vi "test_PhotonPoseEstimator_ClosestToLastfPose.vi"(8 "error in (no error)":errorcluster) -> (0 "error out":errorcluster, 3 "Test Passed":bool)   [LabVIEW 2019]
uses:
  <vilib>/Rock Robotics/WPI/ThirdParty/JAS_Junk/TrajLib/Trajectory_Library.lvlib
  <vilib>/Rock Robotics/WPI/ThirdParty/PhotonVisionLib/PhotonVisionLib.lvlib
  <vilib>/Rock Robotics/WPI/ThirdParty/PhotonVisionLib/Enum/PhotonPoseStrategy_ENUM.ctl
  <vilib>/Rock Robotics/WPI/ThirdParty/JAS_Junk/TrajLib/TypeDef/TRANSLATION3D.ctl
  <vilib>/Rock Robotics/WPI/ThirdParty/JAS_Junk/TrajLib/TypeDef/QUATERNION.ctl
  <vilib>/Rock Robotics/WPI/ThirdParty/JAS_Junk/TrajLib/TypeDef/ROTATION3D.ctl
  <vilib>/Rock Robotics/WPI/ThirdParty/JAS_Junk/TrajLib/TypeDef/POSE3D.ctl
  <vilib>/Rock Robotics/WPI/ThirdParty/PhotonVisionLib/TypeDef/PhotonEstimatedRobotPoseType.ctl
  <vilib>/Rock Robotics/WPI/ThirdParty/PhotonVisionLib/TypeDef/TargetCornerType.ctl
  <vilib>/Rock Robotics/WPI/ThirdParty/JAS_Junk/TrajLib/TypeDef/TRANSFORM3D.ctl
  <vilib>/Rock Robotics/WPI/ThirdParty/PhotonVisionLib/TypeDef/PhotonTrackedTargetType.ctl
panel:
  out "2nd Pos Found":bool
  out "2nd Pose Est":T1={"EstimatedPose"={"Translation3d"={"X"=0.0, "Y"=0.0, "Z"=0.0}, "Rotation3d"={"Q_quaternion"={"R"=1.0, "V"=[0.0, 0.0, 0.0]}}}, "TimeStamp_Seconds"=0.0, "targetsUsed"=[], "Strategy"=enum."LOWEST_AMBIGUITY"} {"targetsUsed"."AltCameraToTarget"."TRANSLATION3D"."Z" format="%14.3f"; "targetsUsed"."AltCameraToTarget"."TRANSLATION3D"."Y" format="%14.3f"; "targetsUsed"."AltCameraToTarget"."TRANSLATION3D"."X" format="%14.3f"; "targetsUsed"."BestCameraToTarget"."TRANSLATION3D"."Z" format="%14.3f"; "targetsUsed"."BestCameraToTarget"."TRANSLATION3D"."Y" format="%14.3f"; "targetsUsed"."BestCameraToTarget"."TRANSLATION3D"."X" format="%14.3f"; "EstimatedPose"."Translation3d"."Z" format="%14.3f"; "EstimatedPose"."Translation3d"."Y" format="%14.3f"; "EstimatedPose"."Translation3d"."X" format="%14.3f"}
  out "1st Pos Found":bool
  out "1st Pose Est":T1={"EstimatedPose"={"Translation3d"={"X"=0.0, "Y"=0.0, "Z"=0.0}, "Rotation3d"={"Q_quaternion"={"R"=1.0, "V"=[0.0, 0.0, 0.0]}}}, "TimeStamp_Seconds"=0.0, "targetsUsed"=[], "Strategy"=enum."LOWEST_AMBIGUITY"} {"targetsUsed"."AltCameraToTarget"."TRANSLATION3D"."Z" format="%14.3f"; "targetsUsed"."AltCameraToTarget"."TRANSLATION3D"."Y" format="%14.3f"; "targetsUsed"."AltCameraToTarget"."TRANSLATION3D"."X" format="%14.3f"; "targetsUsed"."BestCameraToTarget"."TRANSLATION3D"."Z" format="%14.3f"; "targetsUsed"."BestCameraToTarget"."TRANSLATION3D"."Y" format="%14.3f"; "targetsUsed"."BestCameraToTarget"."TRANSLATION3D"."X" format="%14.3f"; "EstimatedPose"."Translation3d"."Z" format="%14.3f"; "EstimatedPose"."Translation3d"."Y" format="%14.3f"; "EstimatedPose"."Translation3d"."X" format="%14.3f"}
  out "Test 0 Passed":bool
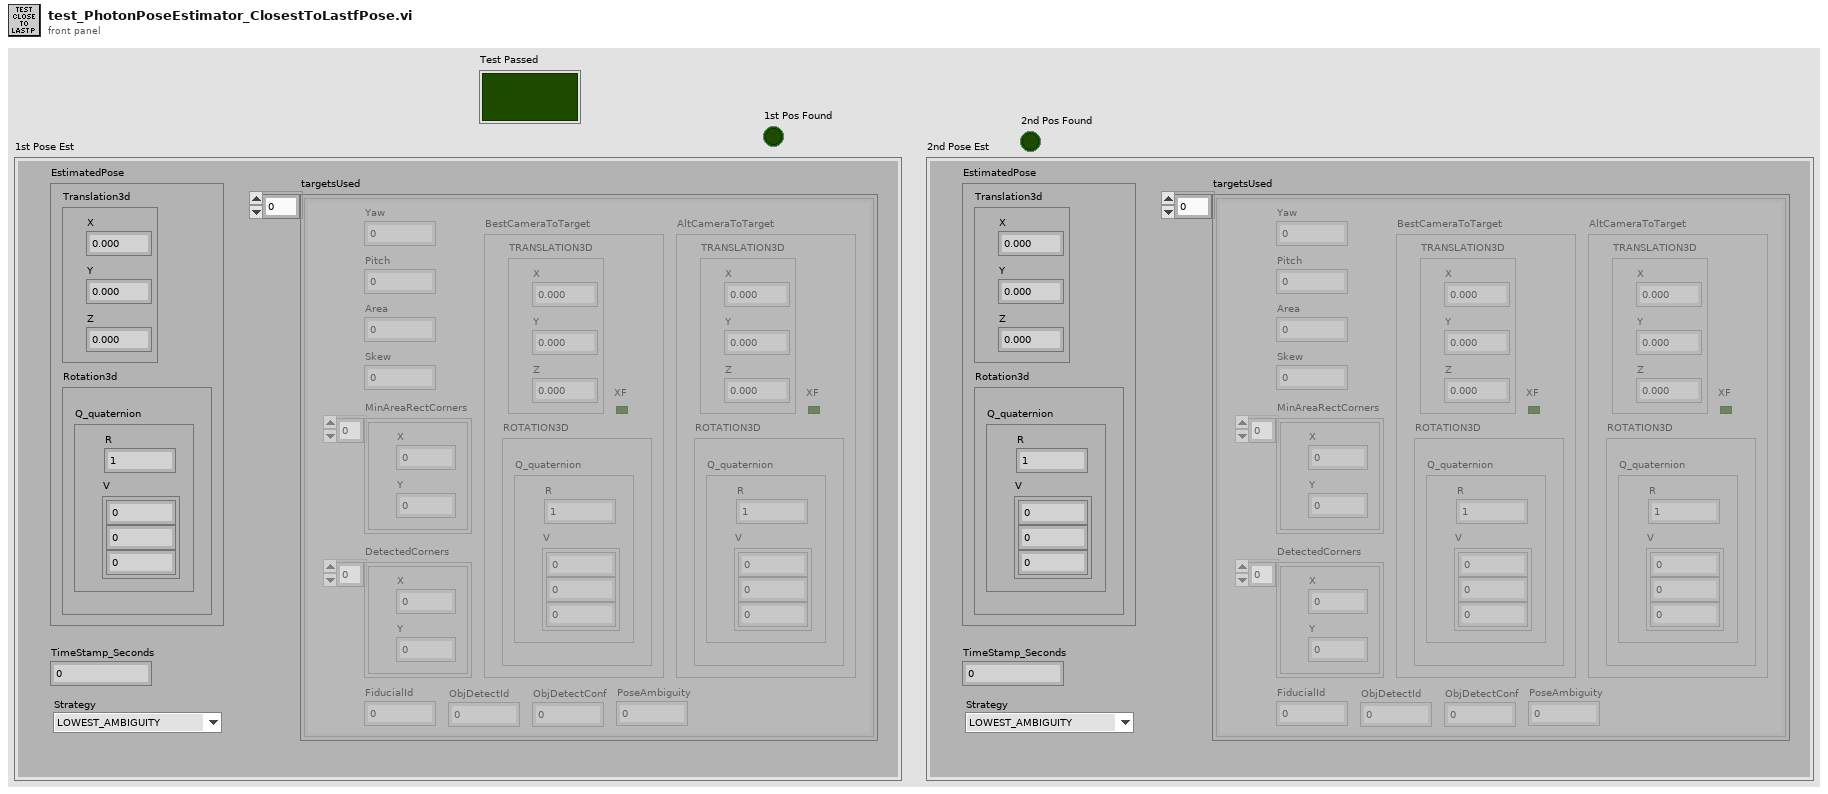
[diagram p1: front panel]
types:
  T1 = typedef "PhotonVisionLib.lvlib/PhotonEstimatedRobotPoseType.ctl" = cluster{"EstimatedPose":T2, "TimeStamp_Seconds":dbl, "targetsUsed":T6[], "Strategy":T9}
  T2 = typedef "Trajectory_Library.lvlib/POSE3D.ctl" = cluster{"Translation3d":T3, "Rotation3d":T4}
  T3 = typedef "Trajectory_Library.lvlib/TRANSLATION3D.ctl" = cluster{"X":dbl, "Y":dbl, "Z":dbl}
  T4 = typedef "Trajectory_Library.lvlib/ROTATION3D.ctl" = cluster{"Q_quaternion":T5}
  T5 = typedef "Trajectory_Library.lvlib/QUATERNION.ctl" = cluster{"R":dbl, "V":dbl[]}
  T6 = typedef "PhotonVisionLib.lvlib/PhotonTrackedTargetType.ctl" = cluster{"Yaw":dbl, "Pitch":dbl, "Area":dbl, "Skew":dbl, "MinAreaRectCorners":T7[], "BestCameraToTarget":T8, "FiducialId":i32, "AltCameraToTarget":T8, "PoseAmbiguity":dbl, "DetectedCorners":T7[], "ObjDetectId":i32, "ObjDetectConf":sgl}
  T7 = typedef "PhotonVisionLib.lvlib/TargetCornerType.ctl" = cluster{"X":dbl, "Y":dbl}
  T8 = typedef "Trajectory_Library.lvlib/TRANSFORM3D.ctl" = cluster{"TRANSLATION3D":T3, "ROTATION3D":T4, "XF":bool}
  T9 = typedef "PhotonVisionLib.lvlib/PhotonPoseStrategy_ENUM.ctl" = enum16{"LOWEST_AMBIGUITY", "CLOSEST_TO_CAMERA_HEIGHT", "CLOSEST_TO_REFERENCE_POSE", "CLOSEST_TO_LAST_POSE", "AVERAGE_BEST_TARGETS", "MULTI_TAG_PNP_ON_COPROCESSOR", "MULTI_TAG_PNP_ON_RIO"}
  T10 = typedef "Trajectory_Library.lvlib/AprilTagFieldLayout.ctl" = cluster{"AprilTagMap":map{i32, T11}, "FieldLength":dbl, "FieldWidth":dbl, "OriginPosition ":T12, "OriginPose3d":T2}
  T11 = typedef "Trajectory_Library.lvlib/AprilTag.ctl" = cluster{"ID":i32, "POSE3D":T2}
  T12 = typedef "Trajectory_Library.lvlib/AprilTagFieldLayoutOrignPosition_ENUM.ctl" = enum16{"kBlueAllianceWallRightSide,", "kRedAllianceWallRightSide,"}
  T13 = typedef "PhotonVisionLib.lvlib/PhotonPipelineMetadataType.ctl" = cluster{"CaptureTimestampMicros":i64, "PublishTimestampMicros":i64, "SequenceID":i64, "TimeSinceLastPong":i64}
  T14 = typedef "PhotonVisionLib.lvlib/PhotonPipelineResultType.ctl" = cluster{"Targets":T6[], "PhotonMultiTargetPNPResult":T15, "PhotonPipelineMetadata":T13}
  T15 = typedef "PhotonVisionLib.lvlib/PhotonMultiTargetPNPResultType.ctl" = cluster{"PhotonPNPResult":T16, "FiducialIDsUsed":i16[]}
  T16 = typedef "PhotonVisionLib.lvlib/PhotonPNPResultType.ctl" = cluster{"IsPresent":bool, "bestReprojErr":dbl, "altReprojErr":dbl, "ambiguity":dbl, "Best":T8, "Alt":T8}
  T17 = typedef "PhotonVisionLib.lvlib/PhotonPoseEstimatorType.ctl" = cluster{"LastPose":T2, "ReferencePose":T2, "FieldTags":T10, "PrimaryStratety":T9, "Camera":string, "RobotToCamera":T8, "ReportedErrors":dbl[], "HighestAmbiguity":dbl, "MultiTagFallbackStrategy":T9, "PoseCacheTimeoutSec":dbl, "PhotonTargetModel":T18, "BaseNTName":string}
  T18 = typedef "PhotonVisionLib.lvlib/PhotonTargetModel.ctl" = cluster{"Vertices":T3[], "IsPlaner":bool, "IsSpherical":bool}
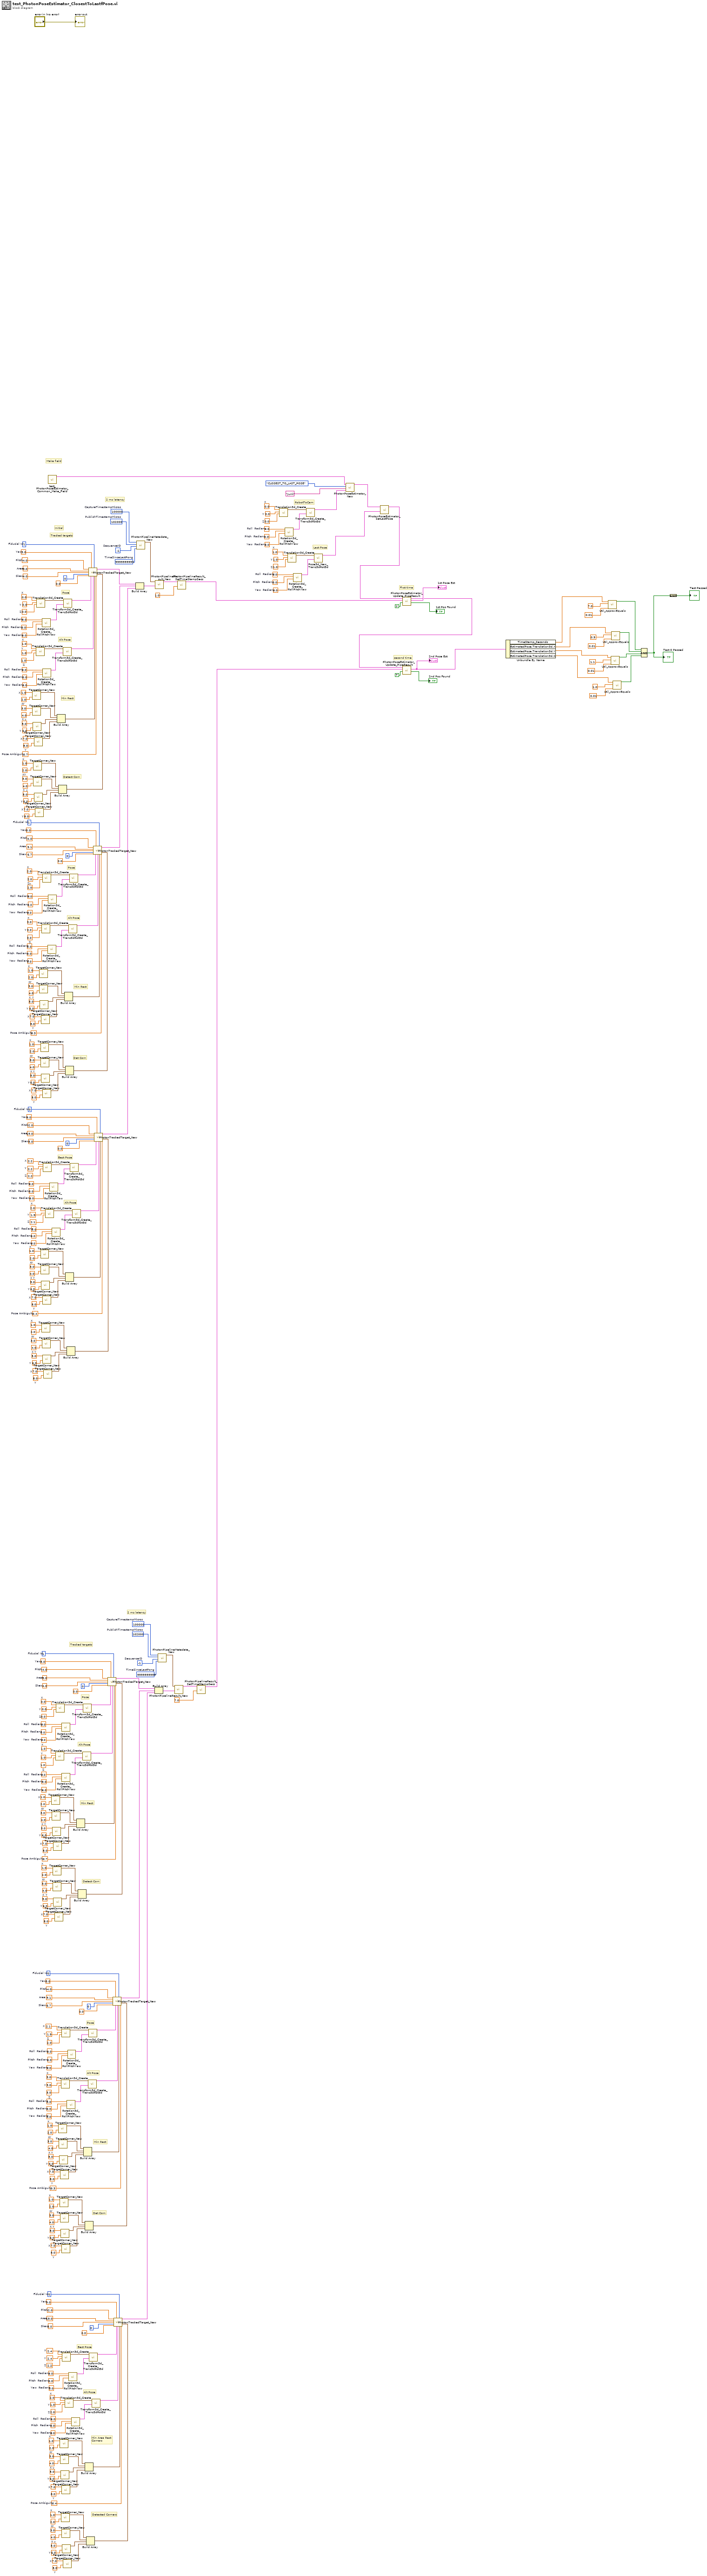
[diagram p0: block diagram]
diagram:
  w15 = i64 100000  # CaptureTimestampMicros
  w16 = i64 102000  # PublishTimestampMicros
  w17 = i64 -1  # SequenceID
  w18 = i64 9999999999  # TimeSinceLastPong
  w20 = i64 100000  # CaptureTimestampMicros
  w21 = i64 102000  # PublishTimestampMicros
  w22 = i64 -1  # SequenceID
  w23 = i64 9999999999  # TimeSinceLastPong
  w46 = 0.0  # Roll  Radians
  w45 = 0.0  # Pitch  Radians
  w44 = 0.0  # Yaw  Radians
  w49 = 2.2  # Z
  w48 = 2.4  # X
  w47 = 2.4  # Y
  w54 = 0.0  # Roll  Radians
  w53 = 0.0  # Pitch  Radians
  w52 = 0.0  # Yaw  Radians
  w57 = 2.0  # Z
  w56 = 2.0  # X
  w55 = 1.0  # Y
  w64 = 7.0  # X
  w65 = 8.0  # Y
  w66 = 5.0  # X
  w67 = 6.0  # Y
  w68 = 3.0  # X
  w69 = 4.0  # Y
  w70 = 1.0  # X
  w71 = 2.0  # Y
  w76 = 7.0  # X
  w77 = 8.0  # Y
  w78 = 5.0  # X
  w79 = 6.0  # Y
  w80 = 3.0  # X
  w81 = 4.0  # Y
  w82 = 1.0  # X
  w83 = 2.0  # Y
  w84 = -2.0  # Pitch
  w85 = 19.0  # Area
  w86 = 3.0  # Skew
  w87 = 0  # Fiducial Id
  w88 = 0.4  # Pose Ambiguity
  w89 = 9.0  # Yaw
  w96 = 0.0  # Roll  Radians
  w95 = 0.0  # Pitch  Radians
  w94 = 0.0  # Yaw  Radians
  w99 = 2.0  # Z
  w98 = 2.1  # X
  w97 = 1.9  # Y
  w104 = 0.0  # Roll  Radians
  w103 = 0.0  # Pitch  Radians
  w102 = 0.0  # Yaw  Radians
  w107 = 3.0  # Z
  w106 = 3.0  # X
  w105 = 3.0  # Y
  w114 = 7.0  # X
  w115 = 8.0  # Y
  w116 = 5.0  # X
  w117 = 6.0  # Y
  w118 = 3.0  # X
  w119 = 4.0  # Y
  w120 = 1.0  # X
  w121 = 2.0  # Y
  w126 = 7.0  # X
  w127 = 8.0  # Y
  w128 = 5.0  # X
  w129 = 6.0  # Y
  w130 = 3.0  # X
  w131 = 4.0  # Y
  w132 = 1.0  # X
  w133 = 2.0  # Y
  w134 = -4.0  # Pitch
  w135 = 9.1  # Area
  w136 = 6.7  # Skew
  w137 = 0  # Fiducial Id
  w138 = 0.3  # Pose Ambiguity
  w139 = 3.0  # Yaw
  w145 = 0.0  # Roll  Radians
  w144 = 0.0  # Pitch  Radians
  w143 = 0.0  # Yaw  Radians
  w148 = 0.0  # Z
  w147 = 0.0  # X
  w146 = 0.0  # Y
  w153 = 0.0  # Roll  Radians
  w152 = 0.0  # Pitch  Radians
  w151 = 0.0  # Yaw  Radians
  w156 = 1.0  # Z
  w155 = 1.0  # X
  w154 = 1.0  # Y
  w163 = 7.0  # X
  w164 = 8.0  # Y
  w165 = 5.0  # X
  w166 = 6.0  # Y
  w167 = 3.0  # X
  w168 = 4.0  # Y
  w169 = 1.0  # X
  w170 = 2.0  # Y
  w175 = 7.0  # X
  w176 = 8.0  # Y
  w177 = 5.0  # X
  w178 = 6.0  # Y
  w179 = 3.0  # X
  w180 = 4.0  # Y
  w181 = 1.0  # X
  w182 = 2.0  # Y
  w183 = -4.0  # Pitch
  w184 = 9.0  # Area
  w185 = 4.0  # Skew
  w186 = 1  # Fiducial Id
  w187 = 0.7  # Pose Ambiguity
  w188 = 3.0  # Yaw
  w194 = 0.0  # Roll  Radians
  w193 = 0.0  # Pitch  Radians
  w192 = 0.0  # Yaw  Radians
  w197 = 1.0  # Z
  w196 = 1.0  # X
  w195 = 1.0  # Y
  w208 = 0.0  # Roll  Radians
  w207 = 0.0  # Pitch  Radians
  w206 = 0.0  # Yaw  Radians
  w211 = 0.0  # Z
  w210 = 0.0  # X
  w209 = 0.0  # Y
  w236 = 0.0  # Roll  Radians
  w235 = 0.0  # Pitch  Radians
  w234 = 0.0  # Yaw  Radians
  w239 = 2.2  # Z
  w238 = 2.2  # X
  w237 = 2.2  # Y
  w244 = 0.0  # Roll  Radians
  w243 = 0.0  # Pitch  Radians
  w242 = 0.0  # Yaw  Radians
  w247 = 2.1  # Z
  w246 = 2.0  # X
  w245 = 1.9  # Y
  w254 = 7.0  # X
  w255 = 8.0  # Y
  w256 = 5.0  # X
  w257 = 6.0  # Y
  w258 = 3.0  # X
  w259 = 4.0  # Y
  w260 = 1.0  # X
  w261 = 2.0  # Y
  w266 = 7.0  # X
  w267 = 8.0  # Y
  w268 = 5.0  # X
  w269 = 6.0  # Y
  w270 = 3.0  # X
  w271 = 4.0  # Y
  w272 = 1.0  # X
  w273 = 2.0  # Y
  w274 = -2.0  # Pitch
  w275 = 19.0  # Area
  w276 = 3.0  # Skew
  w277 = 0  # Fiducial Id
  w278 = 0.4  # Pose Ambiguity
  w279 = 9.0  # Yaw
  w286 = 0.0  # Roll  Radians
  w285 = 0.0  # Pitch  Radians
  w284 = 0.0  # Yaw  Radians
  w289 = 2.0  # Z
  w288 = 2.0  # X
  w287 = 2.0  # Y
  w294 = 0.0  # Roll  Radians
  w293 = 0.0  # Pitch  Radians
  w292 = 0.0  # Yaw  Radians
  w297 = 3.0  # Z
  w296 = 3.0  # X
  w295 = 3.0  # Y
  w304 = 7.0  # X
  w305 = 8.0  # Y
  w306 = 5.0  # X
  w307 = 6.0  # Y
  w308 = 3.0  # X
  w309 = 4.0  # Y
  w310 = 1.0  # X
  w311 = 2.0  # Y
  w316 = 7.0  # X
  w317 = 8.0  # Y
  w318 = 5.0  # X
  w319 = 6.0  # Y
  w320 = 3.0  # X
  w321 = 4.0  # Y
  w322 = 1.0  # X
  w323 = 2.0  # Y
  w324 = -4.0  # Pitch
  w325 = 9.1  # Area
  w326 = 6.7  # Skew
  w327 = 1  # Fiducial Id
  w328 = 0.3  # Pose Ambiguity
  w329 = 3.0  # Yaw
  w336 = 0.0  # Roll  Radians
  w335 = 0.0  # Pitch  Radians
  w334 = 0.0  # Yaw  Radians
  w339 = 0.0  # Z
  w338 = 0.0  # X
  w337 = 0.0  # Y
  w344 = 0.0  # Roll  Radians
  w343 = 0.0  # Pitch  Radians
  w342 = 0.0  # Yaw  Radians
  w347 = 1.0  # Z
  w346 = 1.0  # X
  w345 = 1.0  # Y
  w354 = 7.0  # X
  w355 = 8.0  # Y
  w356 = 5.0  # X
  w357 = 6.0  # Y
  w358 = 3.0  # X
  w359 = 4.0  # Y
  w360 = 1.0  # X
  w361 = 2.0  # Y
  w366 = 7.0  # X
  w367 = 8.0  # Y
  w368 = 5.0  # X
  w369 = 6.0  # Y
  w370 = 3.0  # X
  w371 = 4.0  # Y
  w372 = 1.0  # X
  w373 = 2.0  # Y
  w374 = -4.0  # Pitch
  w375 = 9.0  # Area
  w376 = 4.0  # Skew
  w377 = 1  # Fiducial Id
  w378 = 0.7  # Pose Ambiguity
  w379 = 3.0  # Yaw
  # "2 ms latency"
  # "2 ms latency"
  # "Min Area Rect\nCorners"
  # "Detected Corners"
  # "second time"
  # "First time"
  # "Initial"
  # "Det Corn"
  # "Min Rect"
  # "Pose"
  # "Detect Corn"
  # "Min Rect"
  # "Tracked targets"
  # "Best Pose"
  # "Alt Pose"
  # "Alt Pose"
  # "Pose"
  # "Alt Pose"
  # "Last Pose"
  # "RobotToCam"
  # "Det Corn"
  # "Min Rect"
  # "Pose"
  # "Detect Corn"
  # "Min Rect"
  # "Tracked targets"
  # "Make field"
  # "Best Pose"
  # "Alt Pose"
  # "Alt Pose"
  # "Pose"
  # "Alt Pose"
  n1 = call <vilib>:"TargetCorner_New.vi"("Y"=w373, "X"=w372) -> ("TargetCorner"=w365:T7)  [unwired: 9 in]
  n2 = call <vilib>:"TargetCorner_New.vi"("Y"=w371, "X"=w370) -> ("TargetCorner"=w364:T7)  [unwired: 9 in]
  n3 = call <vilib>:"TargetCorner_New.vi"("Y"=w369, "X"=w368) -> ("TargetCorner"=w363:T7)  [unwired: 9 in]
  n4 = call <vilib>:"TargetCorner_New.vi"("Y"=w361, "X"=w360) -> ("TargetCorner"=w353:T7)  [unwired: 9 in]
  n5 = call <vilib>:"TargetCorner_New.vi"("Y"=w359, "X"=w358) -> ("TargetCorner"=w352:T7)  [unwired: 9 in]
  n6 = call <vilib>:"TargetCorner_New.vi"("Y"=w367, "X"=w366) -> ("TargetCorner"=w362:T7)  [unwired: 9 in]
  n7 = call <vilib>:"TargetCorner_New.vi"("Y"=w357, "X"=w356) -> ("TargetCorner"=w351:T7)  [unwired: 9 in]
  n8 = call <vilib>:"TargetCorner_New.vi"("Y"=w355, "X"=w354) -> ("TargetCorner"=w350:T7)  [unwired: 9 in]
  n9 = call <vilib>:"Translation3d_Create.vi"("Z"=w347, "Y"=w345, "X"=w346) -> ("TRANSLATION3D"=w341:T3)  [unwired: 8 in]
  n10 = call <vilib>:"Translation3d_Create.vi"("Z"=w339, "Y"=w337, "X"=w338) -> ("TRANSLATION3D"=w333:T3)  [unwired: 8 in]
  n11 = call <vilib>:"TargetCorner_New.vi"("Y"=w323, "X"=w322) -> ("TargetCorner"=w315:T7)  [unwired: 9 in]
  n12 = call <vilib>:"TargetCorner_New.vi"("Y"=w321, "X"=w320) -> ("TargetCorner"=w314:T7)  [unwired: 9 in]
  n13 = call <vilib>:"TargetCorner_New.vi"("Y"=w319, "X"=w318) -> ("TargetCorner"=w313:T7)  [unwired: 9 in]
  n14 = call <vilib>:"TargetCorner_New.vi"("Y"=w311, "X"=w310) -> ("TargetCorner"=w303:T7)  [unwired: 9 in]
  n15 = call <vilib>:"TargetCorner_New.vi"("Y"=w273, "X"=w272) -> ("TargetCorner"=w265:T7)  [unwired: 9 in]
  n16 = call <vilib>:"TargetCorner_New.vi"("Y"=w309, "X"=w308) -> ("TargetCorner"=w302:T7)  [unwired: 9 in]
  n17 = call <vilib>:"TargetCorner_New.vi"("Y"=w271, "X"=w270) -> ("TargetCorner"=w264:T7)  [unwired: 9 in]
  n18 = call <vilib>:"TargetCorner_New.vi"("Y"=w317, "X"=w316) -> ("TargetCorner"=w312:T7)  [unwired: 9 in]
  n19 = call <vilib>:"TargetCorner_New.vi"("Y"=w307, "X"=w306) -> ("TargetCorner"=w301:T7)  [unwired: 9 in]
  n20 = call <vilib>:"TargetCorner_New.vi"("Y"=w269, "X"=w268) -> ("TargetCorner"=w263:T7)  [unwired: 9 in]
  n21 = call <vilib>:"Translation3d_Create.vi"("Z"=w297, "Y"=w295, "X"=w296) -> ("TRANSLATION3D"=w291:T3)  [unwired: 8 in]
  n22 = call <vilib>:"TargetCorner_New.vi"("Y"=w261, "X"=w260) -> ("TargetCorner"=w253:T7)  [unwired: 9 in]
  n23 = call <vilib>:"Rotation3d_Create_RollPitchYaw.vi"("Yaw"=w334, "Pitch"=w335, "Roll"=w336) -> ("Rotation3d"=w332:T4)  [unwired: 8 in]
  n24 = call <vilib>:"TargetCorner_New.vi"("Y"=w259, "X"=w258) -> ("TargetCorner"=w252:T7)  [unwired: 9 in]
  n25 = call <vilib>:"Rotation3d_Create_RollPitchYaw.vi"("Yaw"=w342, "Pitch"=w343, "Roll"=w344) -> ("Rotation3d"=w340:T4)  [unwired: 8 in]
  n26 = call <vilib>:"Translation3d_Create.vi"("Z"=w289, "Y"=w287, "X"=w288) -> ("TRANSLATION3D"=w283:T3)  [unwired: 8 in]
  n27 = call <vilib>:"TargetCorner_New.vi"("Y"=w305, "X"=w304) -> ("TargetCorner"=w300:T7)  [unwired: 9 in]
  n28 = call <vilib>:"TargetCorner_New.vi"("Y"=w267, "X"=w266) -> ("TargetCorner"=w262:T7)  [unwired: 9 in]
  n29 = call <vilib>:"TargetCorner_New.vi"("Y"=w257, "X"=w256) -> ("TargetCorner"=w251:T7)  [unwired: 9 in]
  n30 = call <vilib>:"Translation3d_Create.vi"("Z"=w239, "Y"=w237, "X"=w238) -> ("TRANSLATION3D"=w233:T3)  [unwired: 8 in]
  n31 = call <vilib>:"TargetCorner_New.vi"("Y"=w255, "X"=w254) -> ("TargetCorner"=w250:T7)  [unwired: 9 in]
  n32 = call <vilib>:"Translation3d_Create.vi"("Z"=w247, "Y"=w245, "X"=w246) -> ("TRANSLATION3D"=w241:T3)  [unwired: 8 in]
  n33 = call <vilib>:"Rotation3d_Create_RollPitchYaw.vi"("Yaw"=w292, "Pitch"=w293, "Roll"=w294) -> ("Rotation3d"=w290:T4)  [unwired: 8 in]
  n34 = call <vilib>:"Rotation3d_Create_RollPitchYaw.vi"("Yaw"=w284, "Pitch"=w285, "Roll"=w286) -> ("Rotation3d"=w282:T4)  [unwired: 8 in]
  n35 = call "test_PhotonPoseEstimator_Common_Make_Field.vi"() -> ("AprilTagFieldLayout"=w223:T10)  [unwired: 11 in]
  n36 = call <vilib>:"Rotation3d_Create_RollPitchYaw.vi"("Yaw"=w234, "Pitch"=w235, "Roll"=w236) -> ("Rotation3d"=w232:T4)  [unwired: 8 in]
  n37 = call <vilib>:"TargetCorner_New.vi"("Y"=w182, "X"=w181) -> ("TargetCorner"=w174:T7)  [unwired: 9 in]
  n38 = call <vilib>:"Rotation3d_Create_RollPitchYaw.vi"("Yaw"=w242, "Pitch"=w243, "Roll"=w244) -> ("Rotation3d"=w240:T4)  [unwired: 8 in]
  n39 = call <vilib>:"TargetCorner_New.vi"("Y"=w180, "X"=w179) -> ("TargetCorner"=w173:T7)  [unwired: 9 in]
  n40 = call <vilib>:"TargetCorner_New.vi"("Y"=w178, "X"=w177) -> ("TargetCorner"=w172:T7)  [unwired: 9 in]
  n41 = call <vilib>:"TargetCorner_New.vi"("Y"=w170, "X"=w169) -> ("TargetCorner"=w162:T7)  [unwired: 9 in]
  n42 = call <vilib>:"TargetCorner_New.vi"("Y"=w168, "X"=w167) -> ("TargetCorner"=w161:T7)  [unwired: 9 in]
  n43 = call <vilib>:"TargetCorner_New.vi"("Y"=w176, "X"=w175) -> ("TargetCorner"=w171:T7)  [unwired: 9 in]
  n44 = call <vilib>:"TargetCorner_New.vi"("Y"=w166, "X"=w165) -> ("TargetCorner"=w160:T7)  [unwired: 9 in]
  n45 = call <vilib>:"TargetCorner_New.vi"("Y"=w164, "X"=w163) -> ("TargetCorner"=w159:T7)  [unwired: 9 in]
  n46 = call <vilib>:"Translation3d_Create.vi"("Z"=w156, "Y"=w154, "X"=w155) -> ("TRANSLATION3D"=w150:T3)  [unwired: 8 in]
  n47 = call <vilib>:"Translation3d_Create.vi"("Z"=w148, "Y"=w146, "X"=w147) -> ("TRANSLATION3D"=w142:T3)  [unwired: 8 in]
  n48 = Build Array(w365, w364, w363, w362) -> (w349:T7[])
  n49 = Build Array(w353, w352, w351, w350) -> (w348:T7[])
  n50 = call <vilib>:"TargetCorner_New.vi"("Y"=w133, "X"=w132) -> ("TargetCorner"=w125:T7)  [unwired: 9 in]
  n51 = call <vilib>:"TargetCorner_New.vi"("Y"=w131, "X"=w130) -> ("TargetCorner"=w124:T7)  [unwired: 9 in]
  n52 = call <vilib>:"TargetCorner_New.vi"("Y"=w129, "X"=w128) -> ("TargetCorner"=w123:T7)  [unwired: 9 in]
  n53 = call <vilib>:"TargetCorner_New.vi"("Y"=w121, "X"=w120) -> ("TargetCorner"=w113:T7)  [unwired: 9 in]
  n54 = call <vilib>:"TargetCorner_New.vi"("Y"=w83, "X"=w82) -> ("TargetCorner"=w75:T7)  [unwired: 9 in]
  n55 = call <vilib>:"TargetCorner_New.vi"("Y"=w119, "X"=w118) -> ("TargetCorner"=w112:T7)  [unwired: 9 in]
  n56 = call <vilib>:"TargetCorner_New.vi"("Y"=w81, "X"=w80) -> ("TargetCorner"=w74:T7)  [unwired: 9 in]
  n57 = call <vilib>:"TargetCorner_New.vi"("Y"=w127, "X"=w126) -> ("TargetCorner"=w122:T7)  [unwired: 9 in]
  n58 = call <vilib>:"TargetCorner_New.vi"("Y"=w117, "X"=w116) -> ("TargetCorner"=w111:T7)  [unwired: 9 in]
  n59 = call <vilib>:"TargetCorner_New.vi"("Y"=w79, "X"=w78) -> ("TargetCorner"=w73:T7)  [unwired: 9 in]
  n60 = call <vilib>:"Translation3d_Create.vi"("Z"=w107, "Y"=w105, "X"=w106) -> ("TRANSLATION3D"=w101:T3)  [unwired: 8 in]
  n61 = call <vilib>:"TargetCorner_New.vi"("Y"=w71, "X"=w70) -> ("TargetCorner"=w63:T7)  [unwired: 9 in]
  n62 = call <vilib>:"Rotation3d_Create_RollPitchYaw.vi"("Yaw"=w143, "Pitch"=w144, "Roll"=w145) -> ("Rotation3d"=w141:T4)  [unwired: 8 in]
  n63 = call <vilib>:"TargetCorner_New.vi"("Y"=w69, "X"=w68) -> ("TargetCorner"=w62:T7)  [unwired: 9 in]
  n64 = call <vilib>:"Rotation3d_Create_RollPitchYaw.vi"("Yaw"=w151, "Pitch"=w152, "Roll"=w153) -> ("Rotation3d"=w149:T4)  [unwired: 8 in]
  n65 = call <vilib>:"Translation3d_Create.vi"("Z"=w99, "Y"=w97, "X"=w98) -> ("TRANSLATION3D"=w93:T3)  [unwired: 8 in]
  n66 = call <vilib>:"TargetCorner_New.vi"("Y"=w115, "X"=w114) -> ("TargetCorner"=w110:T7)  [unwired: 9 in]
  n67 = call <vilib>:"TargetCorner_New.vi"("Y"=w77, "X"=w76) -> ("TargetCorner"=w72:T7)  [unwired: 9 in]
  n68 = call <vilib>:"TargetCorner_New.vi"("Y"=w67, "X"=w66) -> ("TargetCorner"=w61:T7)  [unwired: 9 in]
  n69 = call <vilib>:"Translation3d_Create.vi"("Z"=w49, "Y"=w47, "X"=w48) -> ("TRANSLATION3D"=w43:T3)  [unwired: 8 in]
  n70 = call <vilib>:"Transform3d_Create_Trans3dRot3d.vi"("Rotation3d"=w340, "Translation3d"=w341) -> ("Transform3d"=w330:T8)  [unwired: 9 in]
  n71 = call <vilib>:"TargetCorner_New.vi"("Y"=w65, "X"=w64) -> ("TargetCorner"=w60:T7)  [unwired: 9 in]
  n72 = call <vilib>:"Transform3d_Create_Trans3dRot3d.vi"("Rotation3d"=w332, "Translation3d"=w333) -> ("Transform3d"=w331:T8)  [unwired: 9 in]
  n73 = Build Array(w315, w314, w313, w312) -> (w299:T7[])
  n74 = call <vilib>:"Translation3d_Create.vi"("Z"=w57, "Y"=w55, "X"=w56) -> ("TRANSLATION3D"=w51:T3)  [unwired: 8 in]
  n75 = Build Array(w303, w302, w301, w300) -> (w298:T7[])
  n76 = Build Array(w265, w264, w263, w262) -> (w249:T7[])
  n77 = Build Array(w253, w252, w251, w250) -> (w248:T7[])
  n78 = call <vilib>:"Rotation3d_Create_RollPitchYaw.vi"("Yaw"=w102, "Pitch"=w103, "Roll"=w104) -> ("Rotation3d"=w100:T4)  [unwired: 8 in]
  n79 = call <vilib>:"Rotation3d_Create_RollPitchYaw.vi"("Yaw"=w94, "Pitch"=w95, "Roll"=w96) -> ("Rotation3d"=w92:T4)  [unwired: 8 in]
  n80 = call <vilib>:"Transform3d_Create_Trans3dRot3d.vi"("Rotation3d"=w290, "Translation3d"=w291) -> ("Transform3d"=w280:T8)  [unwired: 9 in]
  n81 = call <vilib>:"Rotation3d_Create_RollPitchYaw.vi"("Yaw"=w44, "Pitch"=w45, "Roll"=w46) -> ("Rotation3d"=w42:T4)  [unwired: 8 in]
  n82 = call <vilib>:"Transform3d_Create_Trans3dRot3d.vi"("Rotation3d"=w282, "Translation3d"=w283) -> ("Transform3d"=w281:T8)  [unwired: 9 in]
  n83 = call <vilib>:"Transform3d_Create_Trans3dRot3d.vi"("Rotation3d"=w232, "Translation3d"=w233) -> ("Transform3d"=w231:T8)  [unwired: 9 in]
  n84 = call <vilib>:"Rotation3d_Create_RollPitchYaw.vi"("Yaw"=w52, "Pitch"=w53, "Roll"=w54) -> ("Rotation3d"=w50:T4)  [unwired: 8 in]
  n85 = call <vilib>:"Transform3d_Create_Trans3dRot3d.vi"("Rotation3d"=w240, "Translation3d"=w241) -> ("Transform3d"=w230:T8)  [unwired: 9 in]
  n86 = Build Array(w174, w173, w172, w171) -> (w158:T7[])
  n87 = Build Array(w162, w161, w160, w159) -> (w157:T7[])
  n88 = call <vilib>:"Transform3d_Create_Trans3dRot3d.vi"("Rotation3d"=w149, "Translation3d"=w150) -> ("Transform3d"=w140:T8)  [unwired: 9 in]
  n89 = call <vilib>:"Transform3d_Create_Trans3dRot3d.vi"("Rotation3d"=w141, "Translation3d"=w142) -> ("Transform3d"=w9:T8)  [unwired: 9 in]
  n90 = Build Array(w125, w124, w123, w122) -> (w109:T7[])
  n91 = Build Array(w113, w112, w111, w110) -> (w108:T7[])
  n92 = Build Array(w75, w74, w73, w72) -> (w59:T7[])
  n93 = Build Array(w63, w62, w61, w60) -> (w58:T7[])
  n94 = call <vilib>:"Transform3d_Create_Trans3dRot3d.vi"("Rotation3d"=w100, "Translation3d"=w101) -> ("Transform3d"=w90:T8)  [unwired: 9 in]
  n95 = call <vilib>:"PhotonTrackedTarget_New.vi"("Pitch"=w374, "Yaw"=w379, "Fiducial Id"=w377, "Area"=w375, "Skew"=w376, "ObjDetectId"=0, "DetectedCorners"=w348, "DetectObjConf"=sgl 0.0, "BestCameraToTarget"=w331, "AltCameraToTarget"=w330, "MinAreaRectCorners"=w349, "Pose Ambiguity"=w378) -> ("TrackedTarget"=w229:T6)  [unwired: 3 in]
  n96 = call <vilib>:"Transform3d_Create_Trans3dRot3d.vi"("Rotation3d"=w92, "Translation3d"=w93) -> ("Transform3d"=w91:T8)  [unwired: 9 in]
  n97 = call <vilib>:"Transform3d_Create_Trans3dRot3d.vi"("Rotation3d"=w42, "Translation3d"=w43) -> ("Transform3d"=w41:T8)  [unwired: 9 in]
  n98 = call <vilib>:"Transform3d_Create_Trans3dRot3d.vi"("Rotation3d"=w50, "Translation3d"=w51) -> ("Transform3d"=w40:T8)  [unwired: 9 in]
  n99 = call <vilib>:"PhotonTrackedTarget_New.vi"("Pitch"=w324, "Yaw"=w329, "Fiducial Id"=w327, "Area"=w325, "Skew"=w326, "ObjDetectId"=0, "DetectedCorners"=w298, "DetectObjConf"=sgl 0.0, "BestCameraToTarget"=w281, "AltCameraToTarget"=w280, "MinAreaRectCorners"=w299, "Pose Ambiguity"=w328) -> ("TrackedTarget"=w228:T6)  [unwired: 3 in]
  n100 = call <vilib>:"PhotonTrackedTarget_New.vi"("Pitch"=w274, "Yaw"=w279, "Fiducial Id"=w277, "Area"=w275, "Skew"=w276, "ObjDetectId"=0, "DetectedCorners"=w248, "DetectObjConf"=sgl 0.0, "BestCameraToTarget"=w231, "AltCameraToTarget"=w230, "MinAreaRectCorners"=w249, "Pose Ambiguity"=w278) -> ("TrackedTarget"=w227:T6)  [unwired: 3 in]
  n101 = call <vilib>:"PhotonTrackedTarget_New.vi"("Pitch"=w183, "Yaw"=w188, "Fiducial Id"=w186, "Area"=w184, "Skew"=w185, "ObjDetectId"=0, "DetectedCorners"=w157, "DetectObjConf"=sgl 0.0, "BestCameraToTarget"=w9, "AltCameraToTarget"=w140, "MinAreaRectCorners"=w158, "Pose Ambiguity"=w187) -> ("TrackedTarget"=w39:T6)  [unwired: 3 in]
  n102 = call <vilib>:"PhotonTrackedTarget_New.vi"("Pitch"=w134, "Yaw"=w139, "Fiducial Id"=w137, "Area"=w135, "Skew"=w136, "ObjDetectId"=0, "DetectedCorners"=w108, "DetectObjConf"=sgl 0.0, "BestCameraToTarget"=w91, "AltCameraToTarget"=w90, "MinAreaRectCorners"=w109, "Pose Ambiguity"=w138) -> ("TrackedTarget"=w38:T6)  [unwired: 3 in]
  n103 = call <vilib>:"PhotonTrackedTarget_New.vi"("Pitch"=w84, "Yaw"=w89, "Fiducial Id"=w87, "Area"=w85, "Skew"=w86, "ObjDetectId"=0, "DetectedCorners"=w58, "DetectObjConf"=sgl 0.0, "BestCameraToTarget"=w41, "AltCameraToTarget"=w40, "MinAreaRectCorners"=w59, "Pose Ambiguity"=w88) -> ("TrackedTarget"=w24:T6)  [unwired: 3 in]
  n104 = Build Array(w229, w228, w227) -> (w226:T6[])
  n105 = call <vilib>:"PhotonPipelineMetadata_New.vi"("TimeSinceLastPong"=w18, "SequenceID"=w17, "PublishTimestampMicros"=w16, "CaptureTimestampMicros"=w15) -> ("PhotonPipelineMetadata"=w14:T13)  [unwired: 7 in]
  n106 = Build Array(w39, w38, w24) -> (w37:T6[])
  n107 = call <vilib>:"PhotonPipelineResult_New.vi"("TrackedTargets"=w226, "Metadata"=w14) -> ("PhotonPipelineResult"=w225:T14)  [unwired: 9 in]
  n108 = call <vilib>:"PhotonPipelineMetadata_New.vi"("TimeSinceLastPong"=w23, "SequenceID"=w22, "PublishTimestampMicros"=w21, "CaptureTimestampMicros"=w20) -> ("PhotonPipelineMetadata"=w19:T13)  [unwired: 7 in]
  n109 = call <vilib>:"PhotonPipelineResult_New.vi"("TrackedTargets"=w37, "Metadata"=w19) -> ("PhotonPipelineResult"=w36:T14)  [unwired: 9 in]
  n110 = call <vilib>:"PhotonPipelineResult_SetTimeStampSecs.vi"("TimeStampSec"=1.0, "PhotonPipelineResult"=w225) -> ("Out PhotonPipelineResult"=w28:T14)  [unwired: 9 in]
  n111 = call <vilib>:"PhotonPipelineResult_SetTimeStampSecs.vi"("TimeStampSec"=7.0, "PhotonPipelineResult"=w36) -> ("Out PhotonPipelineResult"=w32:T14)  [unwired: 9 in]
  n112 = call <vilib>:"Translation3d_Create.vi"("Z"=w211, "Y"=w209, "X"=w210) -> ("TRANSLATION3D"=w205:T3)  [unwired: 8 in]
  n113 = call <vilib>:"Rotation3d_Create_RollPitchYaw.vi"("Yaw"=w206, "Pitch"=w207, "Roll"=w208) -> ("Rotation3d"=w204:T4)  [unwired: 8 in]
  n114 = call <vilib>:"Translation3d_Create.vi"("Z"=w197, "Y"=w195, "X"=w196) -> ("TRANSLATION3D"=w191:T3)  [unwired: 8 in]
  n115 = call <vilib>:"Rotation3d_Create_RollPitchYaw.vi"("Yaw"=w192, "Pitch"=w193, "Roll"=w194) -> ("Rotation3d"=w190:T4)  [unwired: 8 in]
  n116 = call <vilib>:"Transform3d_Create_Trans3dRot3d.vi"("Rotation3d"=w204, "Translation3d"=w205) -> ("Transform3d"=w203:T8)  [unwired: 9 in]
  n117 = call <vilib>:"Pose3d_New_Trans3dRot3d.vi"("Rotation3d"=w190, "Translation3d"=w191) -> ("outPose3d"=w189:T2)  [unwired: 9 in]
  n118 = call <vilib>:"PhotonPoseEstimator_New.vi"("RobotToCamera"=w203, "Camera"="Junk", "Strategy"=PhotonPoseStrategy_ENUM."CLOSEST_TO_LAST_POSE", "AprilTagFieldLayout"=w223) -> ("PhotonPoseEstimator"=w198:T17)  [unwired: 7 in]
  n119 = call <vilib>:"PhotonPoseEstimator_SetLastPose.vi"("LastPose"=w189, "PhotonPoseEstimator"=w198) -> ("out PhotonPoseEstimator"=w29:T17)  [unwired: 9 in]
  n120 = call <vilib>:"PhotonPoseEstimator_Update_PipeResult.vi"("Has Results"=TRUE, "PipelineResult"=w28, "PhotonPoseEstimator"=w29) -> ("Pos Found"=→"1st Pos Found":bool, "PhotonEstimatedRobotPose"=→"1st Pose Est":T1, "out PhotonPoseEstimator"=w26:T17)  [unwired: 6 in]
  n121 = call <vilib>:"PhotonPoseEstimator_Update_PipeResult.vi"("Has Results"=TRUE, "PipelineResult"=w32, "PhotonPoseEstimator"=w26) -> ("Pos Found"=→"2nd Pos Found":bool, "PhotonEstimatedRobotPose"=w31:T1)  [unwired: 6 in, 1 out]
  "2nd Pose Est" <- w31
  n122 = Unbundle By Name(w31) -> ("TimeStamp_Seconds"=w199:dbl, "EstimatedPose.Translation3d.X"=w214:dbl, "EstimatedPose.Translation3d.Y"=w213:dbl, "EstimatedPose.Translation3d.Z"=w212:dbl)
  n123 = call <vilib>:"Util_ApproxEquals.vi"("Tolerance"=0.01, "Value 2"=7.0, "Value 1"=w199) -> ("ApproxEquals"=w200:bool)  [unwired: 8 in]
  n124 = call <vilib>:"Util_ApproxEquals.vi"("Tolerance"=0.01, "Value 2"=1.1, "Value 1"=w213) -> ("ApproxEquals"=w216:bool)  [unwired: 8 in]
  n125 = call <vilib>:"Util_ApproxEquals.vi"("Tolerance"=0.01, "Value 2"=0.9, "Value 1"=w214) -> ("ApproxEquals"=w382:bool)  [unwired: 8 in]
  n126 = call <vilib>:"Util_ApproxEquals.vi"("Tolerance"=0.01, "Value 2"=1.0, "Value 1"=w212) -> ("ApproxEquals"=w215:bool)  [unwired: 8 in]
  n127 = Compound Arithmetic op=AND(w200, w382, w216, w215) -> (w380:bool)
  "Test 0 Passed" <- w380
  n128 = Compound Arithmetic op=AND(w380) -> (→"Test Passed":bool)
  "error out" <- "error in (no error)"
